vi "Start Sensor.vi"(8 "error in (no error)":errorcluster, 9 "AutoStart?":bool, 10 "Sensor":refnum<class "Sensor.lvclass">, 11 "DemoMain in":refnum<class "DemoMain.lvclass">) -> (0 "error out":errorcluster, 3 "DemoMain out":refnum<class "DemoMain.lvclass">)   [LabVIEW 2012, in "Win8uiDemo.lvlib" / "DemoMain.lvclass"]
uses:
  DemoMain.lvclass
  <vilib>/ActorFramework/Actor/Actor.lvclass
  Sensor Messages/Launch SmallView Msg/Launch SmallView Msg.lvclass
  Sensor Messages/Reschedule Acquire Msg/Reschedule Acquire Msg.lvclass
  Sensor Messages/Request Display Charm Msg/Request Display Charm Msg.lvclass
  Sensor Messages/Launch Detail View Msg/Launch Detail View Msg.lvclass
  Sensor Definition/Sensor.lvclass
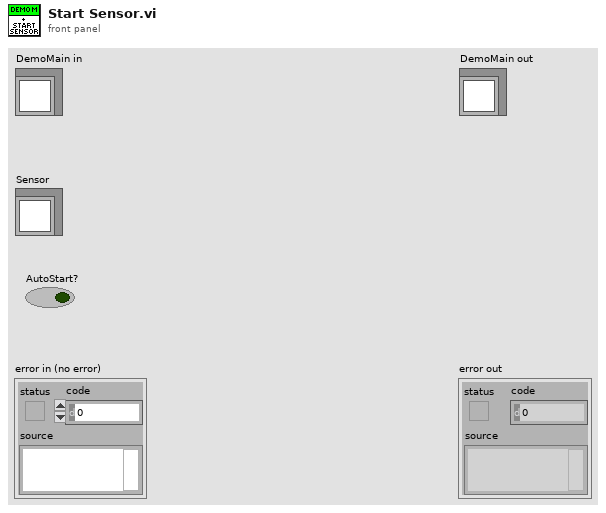
[diagram p1: front panel]
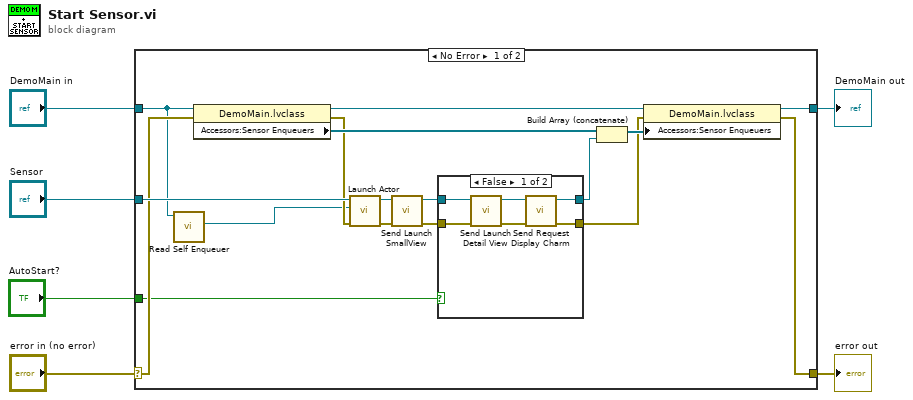
[diagram p0: block diagram]
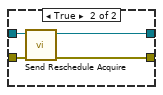
[diagram p2: hidden frame]
diagram:
  n1 = case shown="No Error" "error in (no error)" {
    selector: "error in (no error)" -> [w18 w35]
    tunnel: [w14 w35] -> w5
    tunnel: [w22 w34] -> w3
    tunnel: "DemoMain in" -> [w13 w34]
    tunnel: "Sensor" -> [w23 _]
    tunnel: "AutoStart?" -> [w7 _]
    frame No Error {
      n2 = call <vilib>:"Read Self Enqueuer.vi"("Actor"=w13) -> ("Self Enqueuer"=w12:refnum<class "Message Enqueuer.lvclass">)  [unwired: 10 in]
      n3 = property class="DemoMain.lvclass"(reference=w13, error in=w18) -> (reference out=w21:refnum<class "DemoMain.lvclass">, error out=w17:errorcluster, "Accessors:Sensor Enqueuers"=w20:refnum<class "Message Enqueuer.lvclass">[])
      n4 = call <vilib>:"Launch Actor.vi"("error in (no error)"=w17, "Actor-to-Caller Enqueuer"=w12, "Actor"=w23) -> ("error out"=w15:errorcluster, "Caller-To-Actor Enqueuer"=w16:refnum<class "Message Enqueuer.lvclass">)  [unwired: 7 in]
      n5 = call "Send Launch SmallView.vi"("error in (no error)"=w15, "Message Enqueuer"=w16) -> ("error out"=w9:errorcluster, "Message Enqueuer out"=w11:refnum<class "Message Enqueuer.lvclass">)  [unwired: 8 in]
      n6 = case shown="False" w7 {
        tunnel: w11 -> [w27 w33]
        tunnel: [w29 w32] -> w10
        tunnel: w9 -> [w25 w31]
        tunnel: [w28 w30] -> w8
        frame False {
          n7 = call "Send Launch Detail View.vi"("error in (no error)"=w25, "Message Enqueuer"=w27) -> ("error out"=w24:errorcluster, "Message Enqueuer out"=w26:refnum<class "Message Enqueuer.lvclass">)  [unwired: 8 in]
          n8 = call "Send Request Display Charm.vi"("error in (no error)"=w24, "Message Enqueuer"=w26) -> ("error out"=w28:errorcluster, "Message Enqueuer out"=w29:refnum<class "Message Enqueuer.lvclass">)  [unwired: 8 in]
        }
        frame True {
          n9 = call "Send Reschedule Acquire.vi"("error in (no error)"=w31, "Message Enqueuer"=w33) -> ("error out"=w30:errorcluster, "Message Enqueuer out"=w32:refnum<class "Message Enqueuer.lvclass">)  [unwired: 8 in]
        }
      }
      n10 = Build Array (concatenate)(w20, w10) -> (w19:refnum<class "Message Enqueuer.lvclass">[])
      n11 = property class="DemoMain.lvclass"(reference=w21, error in=w8, "Accessors:Sensor Enqueuers"=w19) -> (reference out=w22:refnum<class "DemoMain.lvclass">, error out=w14:errorcluster)
    }
    frame Error {
    }
  }
  "error out" <- w5
  "DemoMain out" <- w3
